vi "Actor Core.vi"(8 "error in":errorcluster, 11 "Measure Object in":refnum<class "Format Resonances.lvclass">) -> (0 "error out":errorcluster, 3 "Actor out":refnum<class "Actor.lvclass">)   [LabVIEW 2018, in "Format Resonances.lvclass"]
doc: "(<B>Filename</B>: Actor Framework.lvlib:Actor.lvclass:Actor Core.vi)\n\nReceives messages to the actor, reacts to them, and initiates any error handling that may shut the actor down.\n\nDescendant classes may override this VI to append parallel tasks for the actor to complete while it handles messages. Overrides use the Call Parent Method node."
uses:
  Format Resonances.lvclass
  C:/github/LabActor/Template Module/Template Module.lvclass
  C:/Program Files/National Instruments/LabVIEW 2018/vi.lib/ActorFramework/Actor/Actor.lvclass
  <vilib>/ActorFramework/Actor/Actor.lvclass
  Format Resonances Configuration.ctl
  Format Resonances.lvclass/Format Resonances.ctl
  Template Module/Template Module.lvclass/Template Module.ctl
  <vilib>/ActorFramework/Actor/Actor.lvclass/Actor.ctl
  <vilib>/ActorFramework/Message Enqueuer/Message Enqueuer.lvclass/Message Enqueuer.ctl
  NHMFL_Core/Libraries/Instruments/Results/File Path Result/File Path Result.lvclass
  C:/github/NHMFL_Core/Libraries/Instruments/Results/Acquired Result/Acquired Result.lvclass
  Process Object Messages/Process Result Msg/Process Result Msg.lvclass/Process Result Msg.ctl
  Template Module/Read stop event.vi
  <vilib>/ActorFramework/Message Enqueuer/Init from Existing Queue.vi
  <vilib>/ActorFramework/Message Enqueuer/Enqueue.vi
  Process Object Messages/Process Result Msg/Process Result Msg.lvclass
  C:/Program Files/National Instruments/LabVIEW 2018/vi.lib/ActorFramework/Message/Message.lvclass
  <vilib>/ActorFramework/Stop Msg/Stop Msg.lvclass
  <vilib>/ActorFramework/Message Priority Queue/Priority Enqueue.vi
  Process Object/Process Object.lvclass
  <vilib>/ActorFramework/Message Enqueuer/Message Enqueuer.lvclass
panel:
  out "Peak Plot":cluster{"Ramp Pattern":dbl[], "X":dbl[]}[](graph)
  in  "Re-process":bool
  in  "Input file":path
  out "Name":string
  in  "Configuration":T1
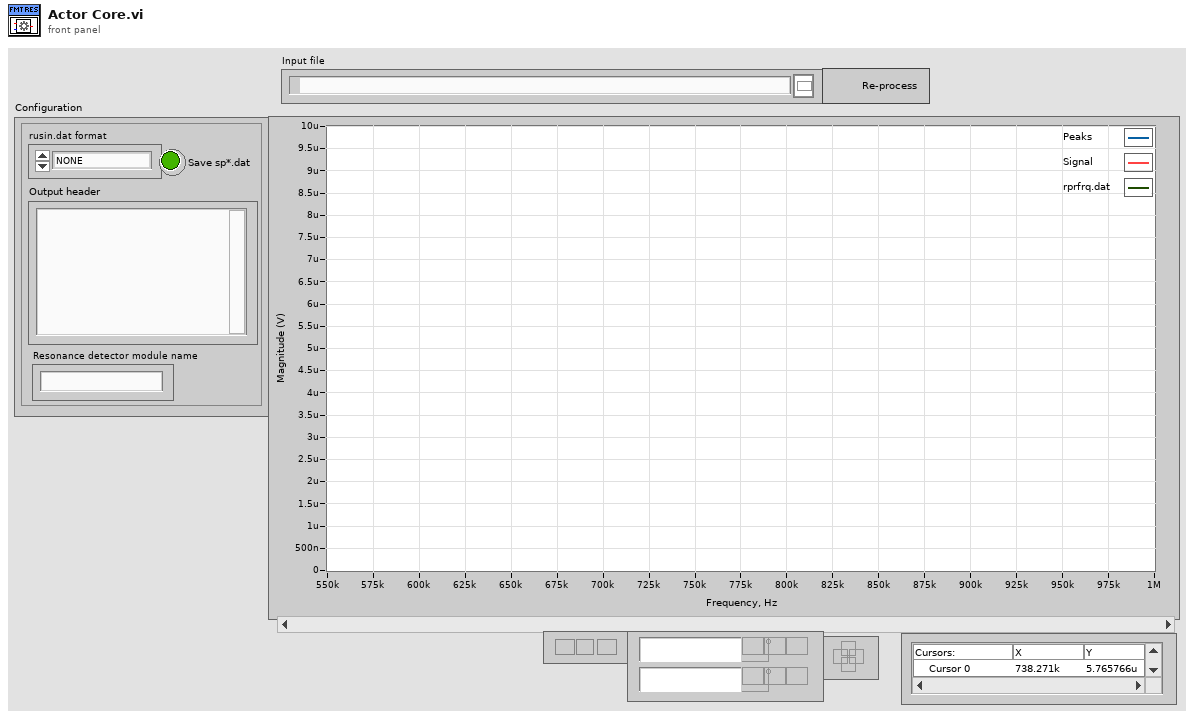
[diagram p1: front panel]
types:
  T1 = typedef "Format Resonances Configuration.ctl" = cluster{"Output header ":string, "rusin\n.dat":enum16{"NONE", "With header", "Without header"}, "Resonance detector module name":string, "Save sp*.dat":bool}
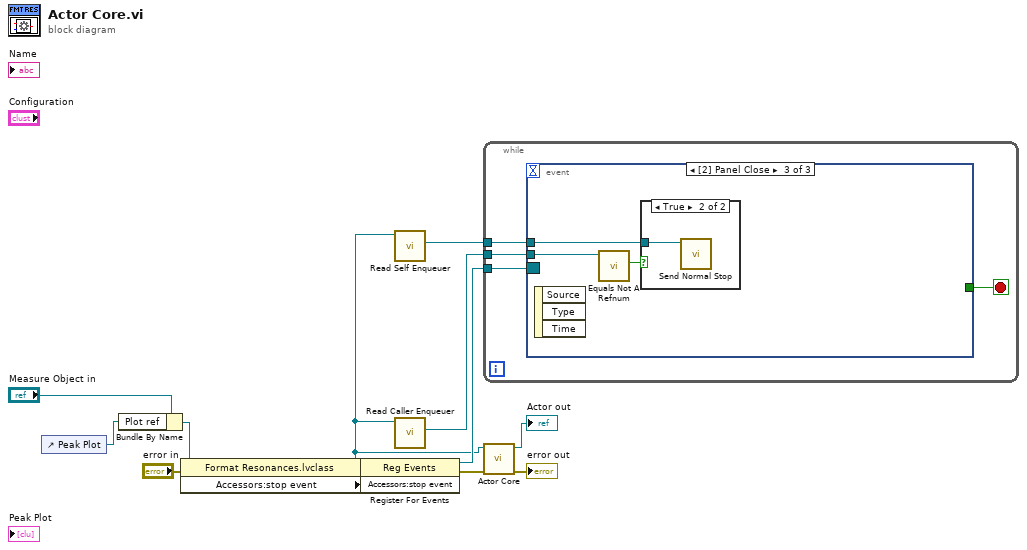
[diagram p0: block diagram]
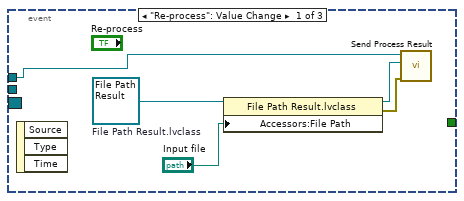
[diagram p2: hidden frame]
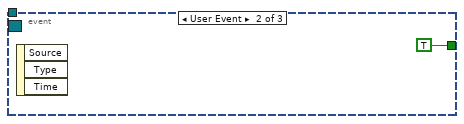
[diagram p3: hidden frame]
diagram:
  n1 = control-ref of="Peak Plot"() -> (w1:refnum<vi>)
  n2 = Bundle By Name(cluster="Measure Object in", "Plot ref"=w1) -> (w2:refnum<class "Format Resonances.lvclass">)
  n3 = property class="Format Resonances.lvclass"(reference=w2, error in="error in") -> (reference out=w4:refnum<class "Format Resonances.lvclass">, error out=w9:errorcluster, "Accessors:stop event"=w11:refnum<user-event>)
  n4 = register-events(error in=w9, w11) -> (reference out=w10:refnum<event-registration>, error out=w3:errorcluster)  [unwired: 1 in]
  n5 = call <vilib>:"Read Self Enqueuer.vi"("Actor"=w4) -> ("Self Enqueuer"=w8:refnum<class "Message Enqueuer.lvclass">)  [unwired: 10 in]
  n6 = call <vilib>:"Read Caller Enqueuer.vi"("Actor"=w4) -> ("Caller Enqueuer"=w7:refnum<class "Message Enqueuer.lvclass">)  [unwired: 10 in]
  n7 = while {
    tunnel: w10 -> [w17]
    tunnel: w8 -> [w15]
    tunnel: w7 -> [w14]
    stop <- w16 stop-if-true
    n8 = event shown="[2] Panel Close" {
      selector: w17 -> [_ _ _]
      dyn-events: _ -> [_ _ _]
      timeout: _ -> [_ _ _]
      tunnel: [_ TRUE _] -> w16
      tunnel: w15 -> [w22 _ w24]
      tunnel: w14 -> [_ _ w26]
      event "Re-process": Value Change {
        w21 = refnum<class "File Path Result.lvclass"> refnum  # File Path Result.lvclass
        n9 = event-data() -> ()  [unwired: 1 in, 3 out]
        n10 = property class="File Path Result.lvclass"(reference=w21, "Accessors:File Path"="Input file") -> (reference out=w20:refnum<class "File Path Result.lvclass">, error out=w19:errorcluster)  [unwired: 1 in]
        n11 = call "Send Process Result.vi"("error in (no error)"=w19, "Result in"=w20, "Message Enqueuer"=w22) -> ()  [unwired: 7 in, 2 out]
      }
      event User Event {
        n12 = event-data() -> ()  [unwired: 1 in, 3 out]
      }
      event Panel Close {
        n13 = event-data() -> ()  [unwired: 1 in, 3 out]
        n14 = call <vilib>:"Equals Not A Refnum.vi"("Message Enqueuer"=w26) -> ("Not a refnum?"=w25:bool)  [unwired: 10 in]
        n15 = case shown="True" w25 {
          tunnel: w24 -> [_ w27]
          frame False {
          }
          frame True {
            n16 = call <vilib>:"Send Normal Stop.vi"("Message Enqueuer"=w27) -> ()  [unwired: 10 in, 1 out]
          }
        }
      }
    }
  }
  n17 = call-parent "Actor Core.vi"("error in"=w3, "Measure Object in"=w4) -> ("error out"=→"error out":errorcluster, "Actor out"=→"Actor out":refnum<class "Actor.lvclass">)  [unwired: 8 in]
